vi "subtract ref wavefront.vi"(8 "error in (no error)":errorcluster, 10 "Slopes file to subtract":path, 11 "HasoSlopes in":refnum<class "HasoSlopes.lvclass">) -> (0 "error out":errorcluster, 3 "HasoSlopes out":refnum<class "HasoSlopes.lvclass">)   [LabVIEW 2020]
uses:
  HasoSlopes.lvclass
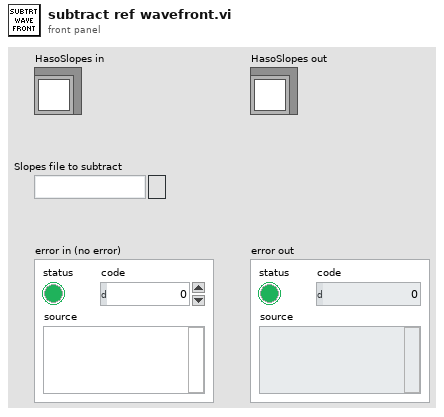
[diagram p1: front panel]
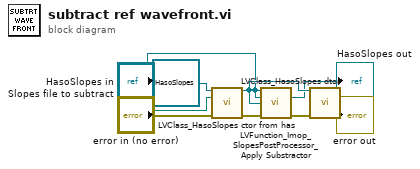
[diagram p0: block diagram]
diagram:
  n1 = call "LVClass_HasoSlopes ctor from has.vi"("HasoSlopes (const)"=refnum<class "HasoSlopes.lvclass"> refnum ("HasoSlopes in"), ".has path"="Slopes file to subtract", "error in (no error)"="error in (no error)") -> ("HasoSlopes (new)"=w9:refnum<class "HasoSlopes.lvclass">, "error out"=w5:errorcluster)  [unwired: 11 in]
  n2 = call "LVFunction_Imop_SlopesPostProcessor_Apply Substractor.vi"("HasoSlopes in"="HasoSlopes in", "HasoSlopes OUT"="HasoSlopes in", "HasoSlopes to substract"=w9, "error in (no error)"=w5) -> ("HasoSlopes OUT 2"=→"HasoSlopes out":refnum<class "HasoSlopes.lvclass">, "error out"=w6:errorcluster)  [unwired: 9 in, 1 out]
  n3 = call "LVClass_HasoSlopes dtor.vi"("HasoSlopes in"=w9, "error in (no error)"=w6) -> ("error out"=→"error out":errorcluster)  [unwired: 12 in, 1 out]
